vi "WaitForState.vi"(8 "error in (no error)":errorcluster, 9 "timeout in ms (-1)":i32=-1 caption="timeout", 10 "State (unknown: any state)":T1 caption="State", 11 "SMO in":refnum<class "SMO.lvclass">) -> (0 "error out":errorcluster, 1 "timed out":bool, 3 "SMO out":refnum<class "SMO.lvclass">)   [LabVIEW 2013, in "SMO.lvclass"]
uses:
  SMO.lvclass
  Typedefs/SMOState --Enum.ctl
  SMO.lvclass/SMO.ctl
  Private/ReftoDVR--SMO.vi
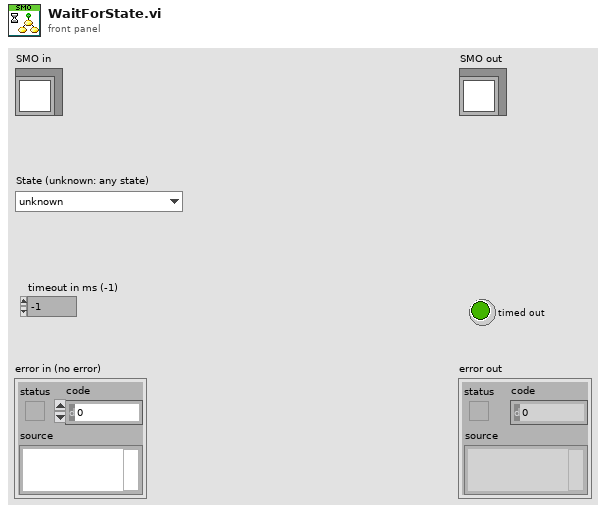
[diagram p1: front panel]
types:
  T1 = typedef "SMO.lvclass/SMOState --Enum.ctl" = enum16{"unknown", "Created", "Started", "Stopped"}
  T2 = typedef "SMO.lvclass/Protected Events.ctl" = cluster{"StopProcesses":refnum<user-event>, "AbortProcesses":refnum<user-event>, "Config Changed":refnum<user-event>, "Dependency":refnum<user-event>}
  T3 = typedef "SMO.lvclass/Public Events.ctl" = cluster{"Error":refnum<user-event>, "State":refnum<user-event>, "Reserve State":refnum<user-event>}
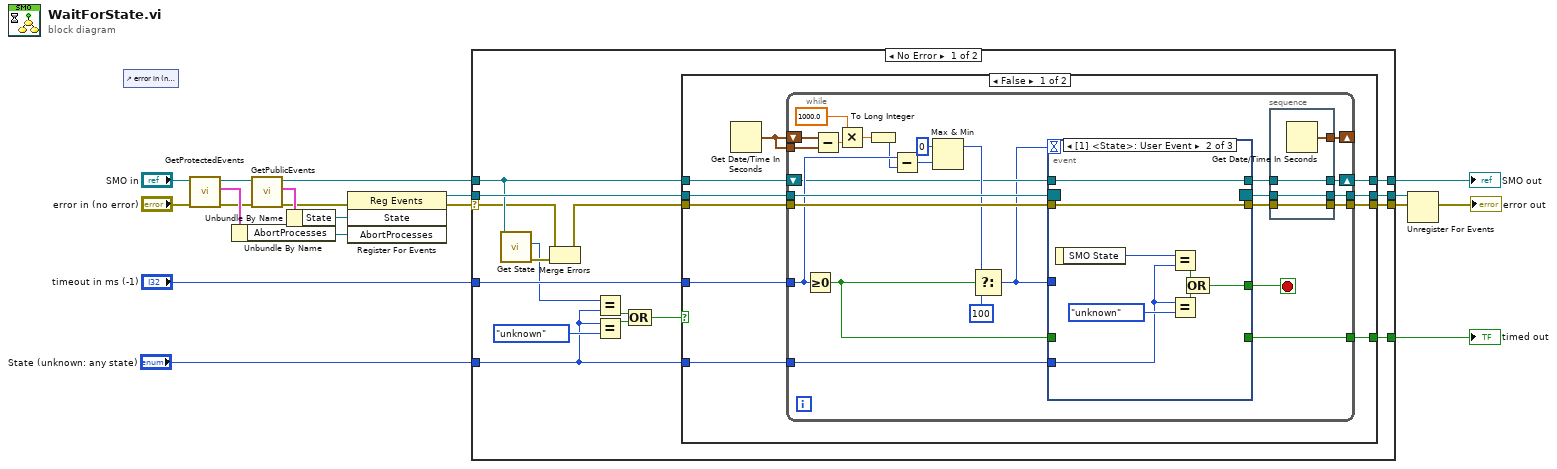
[diagram p0: block diagram]
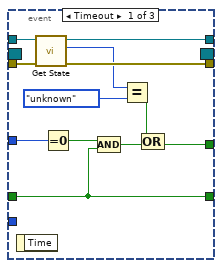
[diagram p2: hidden frame]
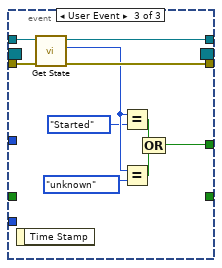
[diagram p3: hidden frame]
diagram:
  n1 = control-ref of="error in (no error)"() -> ()  [unwired: 1 out]
  n2 = call "GetProtectedEvents.vi"("error in (no error)"="error in (no error)", "SMO"="SMO in") -> ("error out"=w6:errorcluster, "SMO Protected Events"=w10:T2, "SMO out"=w8:refnum<class "SMO.lvclass">)  [unwired: 7 in]
  n3 = Unbundle By Name(w10) -> ("AbortProcesses"=w11:refnum<user-event>)
  n4 = call "GetPublicEvents.vi"("error in (no error)"=w6, "SMO"=w8) -> ("error out"=w5:errorcluster, "Public Events"=w9:T3, "SMO out"=w7:refnum<class "SMO.lvclass">)  [unwired: 7 in]
  n5 = Unbundle By Name(w9) -> ("State"=w15:refnum<user-event>)
  n6 = register-events(error in=w5, w15, w11) -> (reference out=w14:refnum<event-registration>, error out=w16:errorcluster)  [unwired: 1 in]
  n7 = case shown="No Error" w16 {
    selector: w16 -> [w27 w111]
    tunnel: [w35 w111] -> w2
    tunnel: w14 -> [w34 w110]
    tunnel: "timeout in ms (-1)" -> [w33 _]
    tunnel: [w32 w110] -> w17
    tunnel: "State (unknown: any state)" -> [w21 _]
    tunnel: [w31 _] -> w13
    tunnel: w7 -> [w29 w109]
    tunnel: [w30 w109] -> w12
    frame No Error {
      n8 = call "Get State.vi"("SMO"=w29) -> ("error out"=w28:errorcluster, "SMO State"=w22:T1)  [unwired: 8 in, 1 out]
      n9 = Merge Errors(w27, w28) -> (w26:errorcluster)
      n10 = Equal?(x=w22, y=w21) -> (x = y?=w24:bool)
      n11 = Equal?(x=w21, y=SMOState_--Enum."unknown") -> (x = y?=w25:bool)
      n12 = Compound Arithmetic op=OR(w24, w25) -> (w20:bool)
      n13 = case shown="False" w20 {
        tunnel: [w45 w106] -> w35
        tunnel: w34 -> [w44 w107]
        tunnel: w33 -> [w43 _]
        tunnel: [w42 w107] -> w32
        tunnel: [w41 _] -> w31
        tunnel: [w40 w108] -> w30
        tunnel: w29 -> [w38 w108]
        tunnel: w26 -> [w37 w106]
        tunnel: w21 -> [w36 _]
        frame False {
          n14 = Get Date/Time In Seconds() -> (seconds since 1Jan1904=w39:timestamp)
          n15 = while {
            tunnel: [w48] -> w45
            tunnel: w44 -> [w71]
            tunnel: w37 -> [w70]
            tunnel: w43 -> [w59]
            tunnel: [w49] -> w42
            tunnel: w36 -> [w69]
            shift-right: [w63] -> _
            shift-left: w39 -> [w62]
            tunnel: [w65] -> w41
            shift-right: [w51] -> w40
            shift-left: w38 -> [w54]
            tunnel: w39 -> [w61]
            stop <- w46 stop-if-true
            n16 = Greater Or Equal To 0?(x=w59) -> (x >= 0?=w64:bool)
            n17 = Subtract(x=w62, y=w61) -> (x-y=w60:dbl)
            n18 = Multiply(x=1000.0 ("timeout in ms (-1)"), y=w60) -> (x*y=w66:dbl)
            n19 = To Long Integer(number=w66) -> (32bit integer=w58:i32)
            n20 = Subtract(x=w59, y=w58) -> (x-y=w57:i32)
            n21 = Max & Min(x=0, y=w57) -> (max(x,y)=w55:i32)  [unwired: 1 out]
            n22 = Select(t=w55, s=w64, f=100 ("timeout in ms (-1)")) -> (s? t:f=w53:i32)
            n23 = event shown="[1] <State>: User Event" {
              selector: w71 -> [_ _ _]
              dyn-events: [_ _ _] -> w50
              timeout: w53 -> [_ _ _]
              tunnel: w70 -> [w83 w95 w103]
              tunnel: [w82 w95 w102] -> w47
              tunnel: [w85 w88 w96] -> w46
              tunnel: w69 -> [_ w90 _]
              tunnel: [w76 _ _] -> w65
              tunnel: w64 -> [w76 _ _]
              tunnel: w53 -> [w78 _ _]
              tunnel: w54 -> [w87 w89 w105]
              tunnel: [w86 w89 w104] -> w52
              event Timeout {
                n24 = event-data() -> ()  [unwired: 1 in, 1 out]
                n25 = call "Get State.vi"("error in (no error)"=w83, "SMO"=w87) -> ("error out"=w82:errorcluster, "SMO State"=w80:T1, "SMO out"=w86:refnum<class "SMO.lvclass">)  [unwired: 7 in]
                n26 = Equal To 0?(x=w78) -> (x = 0?=w77:bool)
                n27 = Compound Arithmetic op=AND(w77, w76) -> (w79:bool)
                n28 = Equal?(x=w80, y=SMOState_--Enum."unknown") -> (x = y?=w84:bool)
                n29 = Compound Arithmetic op=OR(w84, w79) -> (w85:bool)
              }
              event User Event {
                n30 = event-data() -> ("SMO State"=w92:T1)  [unwired: 1 in]
                n31 = Equal?(x=w92, y=w90) -> (x = y?=w93:bool)
                n32 = Equal?(x=w90, y=SMOState_--Enum."unknown") -> (x = y?=w94:bool)
                n33 = Compound Arithmetic op=OR(w93, w94) -> (w88:bool)
              }
              event User Event {
                n34 = event-data() -> ()  [unwired: 1 in, 1 out]
                n35 = call "Get State.vi"("error in (no error)"=w103, "SMO"=w105) -> ("error out"=w102:errorcluster, "SMO State"=w100:T1, "SMO out"=w104:refnum<class "SMO.lvclass">)  [unwired: 7 in]
                n36 = Equal?(x=w100, y=SMOState_--Enum."Started") -> (x = y?=w98:bool)
                n37 = Equal?(x=w100, y=SMOState_--Enum."unknown") -> (x = y?=w97:bool)
                n38 = Compound Arithmetic op=OR(w98, w97) -> (w96:bool)
              }
            }
            n39 = stacked-sequence {
              tunnel: [w75] -> w63
              tunnel: w52 -> [w74]
              tunnel: [w74] -> w51
              tunnel: w50 -> [w73]
              tunnel: [w73] -> w49
              tunnel: [w72] -> w48
              tunnel: w47 -> [w72]
              frame #0 {
                n40 = Get Date/Time In Seconds() -> (seconds since 1Jan1904=w75:timestamp)
              }
            }
          }
        }
        frame True {
          # "Condition already satisfied.\nDo not wait for state transition"
        }
      }
    }
    frame Error {
    }
  }
  "SMO out" <- w12
  "timed out" <- w13
  n41 = Unregister For Events(event registration refnum=w17, error in=w2) -> (error out=→"error out":errorcluster)
